vi "MoveXY.vi"(2 "Iterations":i32, 3 "Current":cluster{dbl, dbl}, 4 "Desired":cluster{"left":i16, "top":i16}, 5 "Map in":refnum<vi>) -> (0 "Final location":cluster{"left":i16, "top":i16}, 1 "Map out":refnum<vi>)   [LabVIEW 2012]
panel:
  out "x/y 2":cluster{dbl, dbl}
  out "x/y":cluster{dbl, dbl}
  # "`"
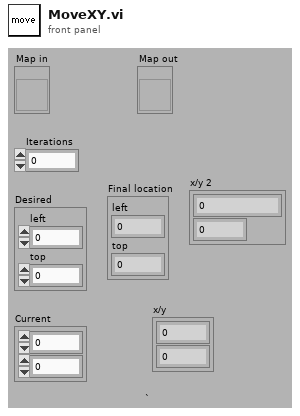
[diagram p1: front panel]
types:
  T1 = typedef "LVPointTypeDef.ctl" = cluster{"Horizontal":i16, "Vertical":i16}
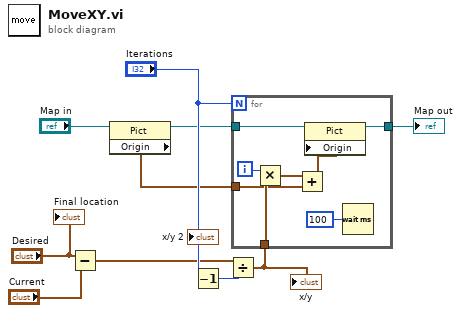
[diagram p0: block diagram]
diagram:
  n1 = Subtract(x="Desired", y="Current") -> (x-y=w5:cluster{dbl, dbl})
  n2 = property class="Pict"(reference="Map in") -> (reference out=w1:refnum<vi>, "Origin"=w2:T1)  [unwired: 1 in, 1 out]
  n3 = Decrement(x="Iterations") -> (x-1=w8:i32)
  n4 = Divide(x=w5, y=w8) -> (x/y=w6:cluster{dbl, dbl})
  "x/y" <- w6
  n5 = for {
    N: "Iterations" -> [_]
    tunnel: w1 -> [w18]
    tunnel: [w17] -> w4
    tunnel: w6 -> [w14]
    tunnel: w2 -> [w11]
    i -> [w15]
    n6 = Multiply(x=w15, y=w14) -> (x*y=w16:cluster{dbl, dbl})
    n7 = Add(x=w16, y=w11) -> (x+y=w12:cluster{dbl, dbl})
    n8 = property class="Pict"(reference=w18, "Origin"=w12) -> (reference out=w17:refnum<vi>)  [unwired: 1 in, 1 out]
    n9 = Wait (ms)(milliseconds to wait=u32 100) -> ()  [unwired: 1 out]
  }
  "Map out" <- w4
  "Final location" <- "Desired"
